vi "MHM Get Cal Data.vi"(8 "error in (no error)":errorcluster, 9 "pulNumberOfBytes":u32, 10 "ulParam":u32, 11 "ulMHMHandle":u32) -> (0 "error out":errorcluster, 1 "plData":i32[](array[numeric]), 2 "pulNumberOfBytes out":u32, 3 "function return":u32)   [LabVIEW 2019, in "MHM_1SL_interface.lvlib"]
uses:
  MHM_1SL_interface.lvlib
  lib/MHM_1SL_interface.dll
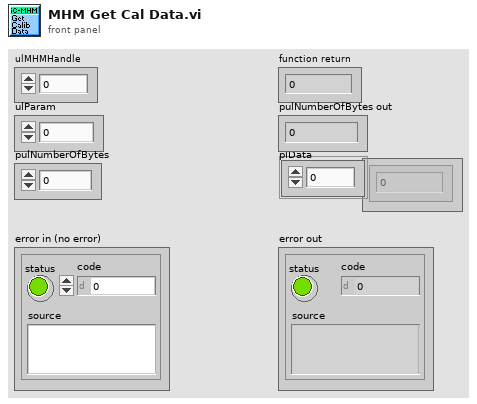
[diagram p1: front panel]
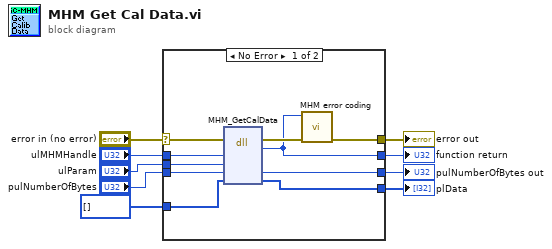
[diagram p0: block diagram]
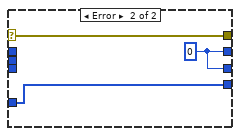
[diagram p2: hidden frame]
diagram:
  n1 = case shown="No Error" "error in (no error)" {
    selector: "error in (no error)" -> [w19 w22]
    tunnel: "ulMHMHandle" -> [w18 _]
    tunnel: [w16 w22] -> w7
    tunnel: [w15 w20] -> w6
    tunnel: i32[] [] ("plData") -> [w14 w21]
    tunnel: [w11 w21] -> w4
    tunnel: "pulNumberOfBytes" -> [w13 _]
    tunnel: "ulParam" -> [w12 _]
    tunnel: [w10 w20] -> w1
    frame No Error {
      n2 = dll-call lib="C:/workspace/project/scancon/MHM_1SL_interface_4.4.0/lv_interface/lib/MHM_1SL_interface.dll" fn="MHM_GetCalData"(error in=w19, "ulMHMHandle"=w18, "ulParam"=w12, "pulNumberOfBytes"=w13, "plData"=w14) -> (error out=w17:errorcluster, "return type"=w15:u32, "pulNumberOfBytes"=w10:u32, "plData"=w11:i32[])  [unwired: 4 in, 1 out]
      n3 = call "MHM error coding.vi"("error in (no error)"=w17, "function return in"=w15) -> ("error out"=w16:errorcluster)  [unwired: 9 in]
    }
    frame Error {
      w20 = u32 0
    }
  }
  "function return" <- w6
  "error out" <- w7
  "plData" <- w4
  "pulNumberOfBytes out" <- w1
